vi "PID_Planta_openloop.vi"() -> ()   [LabVIEW 2010]
panel:
  in  "umanual":dbl(slide) scale=0.0..10.0
  in  "dt":dbl=0.1
  out "Nivel":dbl(slide)=0.1 scale=0.0..0.2
  in  "stop":bool
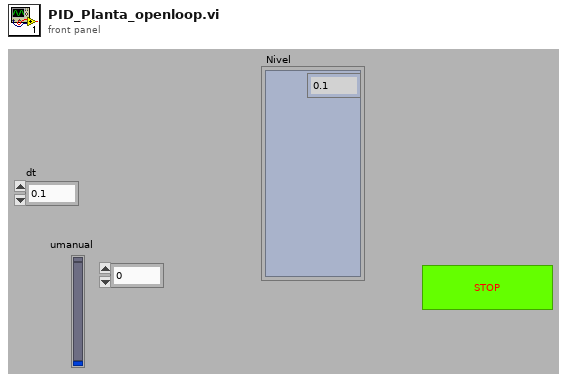
[diagram p1: front panel]
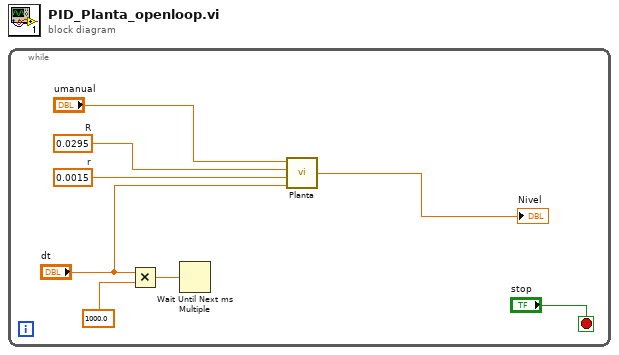
[diagram p0: block diagram]
diagram:
  n1 = while {
    stop <- "stop" stop-if-true
    w1 = 0.0015  # r
    w2 = 0.0295  # R
    n2 = Multiply(x="dt", y=1000.0) -> (x*y=w6:dbl)
    n3 = Wait Until Next ms Multiple(millisecond multiple=w6) -> ()  [unwired: 1 out]
    n4 = call "Planta.vi"("u"="umanual", "R"=w2, "r"=w1, "dt"="dt") -> ("h"=→"Nivel":dbl)  [unwired: 1 in]
  }
